vi "Sprite_ReadValue.vi"(11 "Address":u32) -> (3 "Value":u8)   [LabVIEW 2020]
uses:
  <vilib>/Utility/file.llb/Application Directory.vi
  <vilib>/picture/bmp.llb/Read BMP File.vi
  <vilib>/rvi/DataTransferAndStorage/Container/XNode/niFpgaContainer.xnode
  <vilib>/rvi/Memory/Memory_Emulation/nirvimemoryFastEmulation.vi
  <vilib>/rvi/Memory/Memory_Emulation/nirvimemoryEmulation.vi
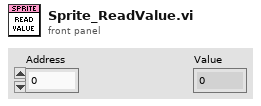
[diagram p1: front panel]
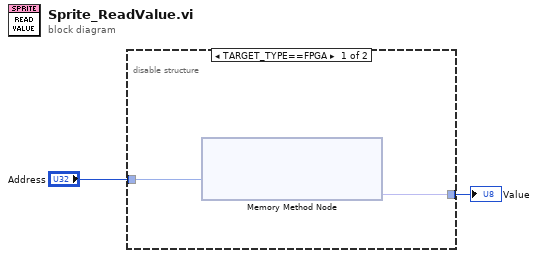
[diagram p0: block diagram]
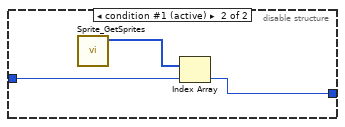
[diagram p2: hidden frame]
diagram:
  n1 = disable-structure shown="TARGET_TYPE==FPGA" {
    disable-tunnel: "Address" -> [w4 w7]
    disable-tunnel: [w3 w6] -> w2
    frame condition #0 {
      n2 = xnode ("Memory Method Node")("Address"=w4) -> ("Data"=w3:fxp<+,6,6>)  [unwired: 1 in, 1 out]
    }
    frame condition #1 (active) {
      n3 = call "Sprite_GetSprites.vi"() -> ("Sprites"=w5:u8[])  [unwired: 11 in]
      n4 = Index Array(array=w5, index=w7) -> (element=w6:u8)
    }
  }
  "Value" <- w2
